vi "Read OffsetDef.lvclass.vi"(8 "error in (no error)":errorcluster, 11 "Offset.lvclass in":refnum<class "Offset.lvclass">) -> (0 "error out":errorcluster, 2 "OffsetDef.lvclass":refnum<class "OffsetDef.lvclass">, 3 "Offset.lvclass out":refnum<class "Offset.lvclass">)   [LabVIEW 2022 SP3, in "TCSDataDefinitions.lvlib" / "TCSCommand.lvlib" / "OffsetCommands.lvlib" / "Offset.lvclass"]
uses:
  Offset.lvclass
  OffsetDef/OffsetDef/OffsetDef.lvclass
  Offset.lvclass/Offset.ctl
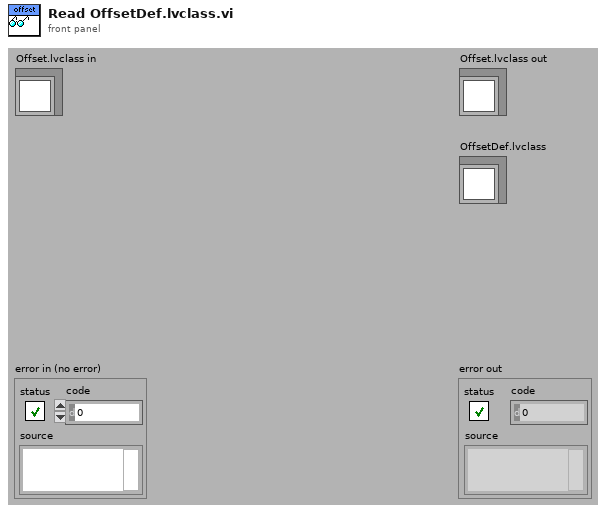
[diagram p1: front panel]
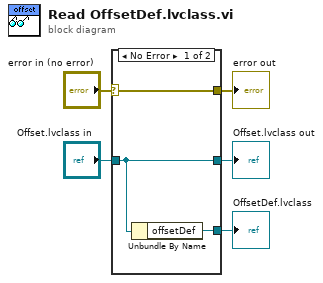
[diagram p0: block diagram]
diagram:
  n1 = case shown="No Error" "error in (no error)" {
    selector: "error in (no error)" -> [w8 w9]
    tunnel: [w8 w9] -> w4
    tunnel: [w7 w10] -> w2
    tunnel: "Offset.lvclass in" -> [w7 w10]
    tunnel: [w6 _] -> w1
    frame No Error {
      n2 = Unbundle By Name(w7) -> ("offsetDef"=w6:refnum<class "OffsetDef.lvclass">)
    }
    frame Error {
    }
  }
  "error out" <- w4
  "Offset.lvclass out" <- w2
  "OffsetDef.lvclass" <- w1
